vi "Resize Image (WxH).vi"(7 "Filter (Default)":T1, 8 "error in (no error)":errorcluster, 9 "Height":i32, 10 "Width":i32, 11 "Image":T2) -> (0 "error out":errorcluster, 3 "Resized Image":T2)   [LabVIEW 2020, in "G-Image.lvlib"]
doc: "Resize the input image to the specified width and height.\n\n<b>Filter</b> sets the filter type used when resizing. When set to Default, the Catmull-Rom filter is used when upsampling images, and the Mitchell filter used when downsampling images.\n\n<b>Note:</b> 8-bit images will be converted to true color images when resized."
uses:
  G-Image.lvlib
  <vilib>/picture/picture.llb/imagedata.ctl
  Controls/Resize Filter.ctl
  <vilib>/Utility/error.llb/Error Cluster From Error Code.vi
  lib/g_image_32.dll
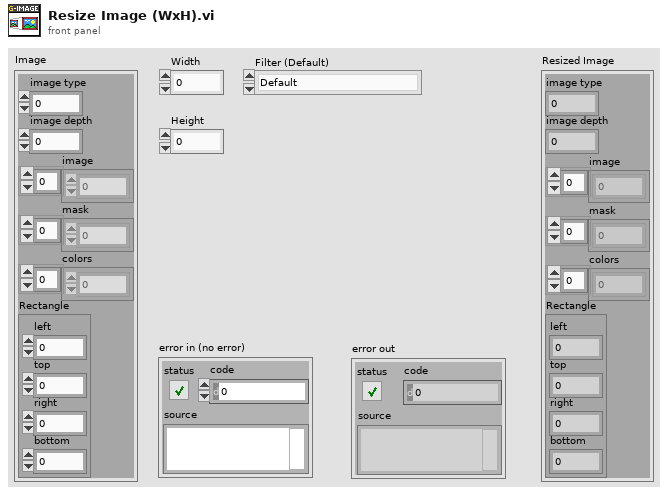
[diagram p1: front panel]
types:
  T1 = typedef "G-Image.lvlib/Resize Filter.ctl" = enum16{"Default", "Box", "Triangle", "Cubic B-Spline", "Catmull-Rom", "Mitchell"}
  T2 = typedef "imagedata.ctl" = cluster{"image type":i32, "image depth":i32, "image":u8[], "mask":u8[], "colors":u32[], "Rectangle":cluster{"left":i16, "top":i16, "right":i16, "bottom":i16}}
  T3 = cluster{"left":i16, "top":i16, "right":i16, "bottom":i16}
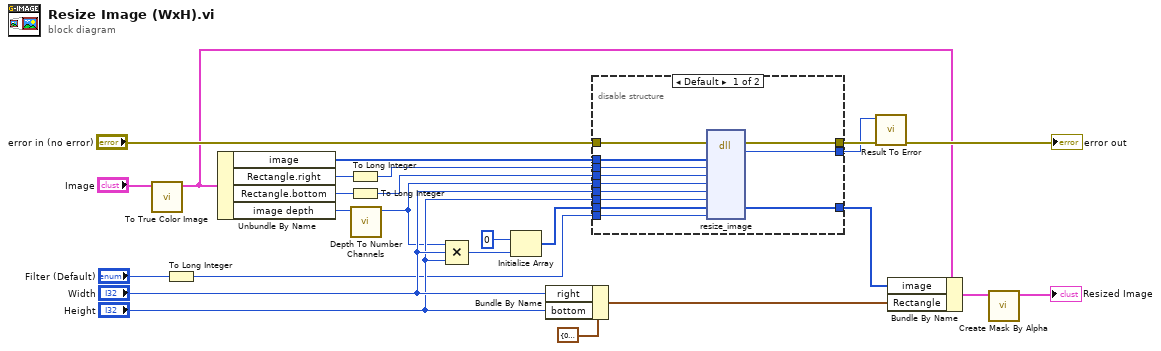
[diagram p0: block diagram]
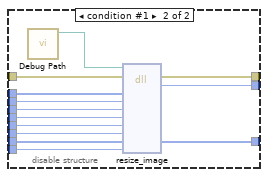
[diagram p2: hidden frame]
diagram:
  n1 = call "To True Color Image.vi"("Image"="Image") -> ("True Color Image"=w3:T2)  [unwired: 9 in, 1 out]
  n2 = To Long Integer(number="Filter (Default)") -> (32bit integer=w1:i32)
  n3 = Unbundle By Name(w3) -> ("image"=w25:u8[], "Rectangle.right"=w12:i16, "Rectangle.bottom"=w10:i16, "image depth"=w6:i32)
  n4 = To Long Integer(number=w12) -> (32bit integer=w11:i32)
  n5 = To Long Integer(number=w10) -> (32bit integer=w9:i32)
  n6 = call "Depth To Number Channels.vi"("Depth"=w6) -> ("Channels"=w5:i32)  [unwired: 10 in]
  n7 = Compound Arithmetic op=MULTIPLY(w5, "Width", "Height") -> (w23:i32)
  n8 = Initialize Array(u8 0, w23) -> (w15:u8[])
  n9 = Bundle By Name(cluster=T3 {"left"=0, "top"=0, "right"=0, "bottom"=0} ("Rectangle"), "right"="Width", "bottom"="Height") -> (w19:T3)
  n10 = disable-structure shown="Default" {
    disable-tunnel: [w37 w50] -> w18
    disable-tunnel: "error in (no error)" -> [w36 w49]
    disable-tunnel: [w35 w48] -> w17
    disable-tunnel: w25 -> [w34 w47]
    disable-tunnel: w11 -> [w33 w46]
    disable-tunnel: w9 -> [w32 w45]
    disable-tunnel: w5 -> [w31 w44]
    disable-tunnel: "Width" -> [w30 w43]
    disable-tunnel: "Height" -> [w29 w42]
    disable-tunnel: w15 -> [w28 w41]
    disable-tunnel: [w27 w40] -> w14
    disable-tunnel: w1 -> [w26 w38]
    frame condition #0 (active) {
      n11 = dll-call lib="C:/github/dataflowg/g-image/src/LabVIEW/G-Image/lib/g_image_*.*" fn="resize_image"(error in=w36, "image_data_in"=w34, "width_in"=w33, "height_in"=w32, "channels_in"=w31, "width_resize"=w30, "height_resize"=w29, "image_data_out"=w28, "filter"=w26) -> (error out=w37:errorcluster, "result"=w35:i32, "image_data_out"=w27:u8[])  [unwired: 9 in, 1 out]
    }
    frame condition #1 {
      n12 = call "Debug Path.vi"() -> ("Debug Path"=w39:path)  [unwired: 11 in]
      n13 = dll-call lib="?" fn="resize_image"(path in=w39, error in=w49, "image_data_in"=w47, "width_in"=w46, "height_in"=w45, "channels_in"=w44, "width_resize"=w43, "height_resize"=w42, "image_data_out"=w41, "filter"=w38) -> (error out=w50:errorcluster, "result"=w48:i32, "image_data_out"=w40:u8[])  [unwired: 8 in, 1 out]
    }
  }
  n14 = call "Result To Error.vi"("error in (no error)"=w18, "Result Code"=w17) -> ("error out"=→"error out":errorcluster)  [unwired: 9 in]
  n15 = Bundle By Name(cluster=w3, "image"=w14, "Rectangle"=w19) -> (w8:T2)
  n16 = call <vilib>:"Create Mask By Alpha.vi"("image data"=w8) -> ("masked image data"=→"Resized Image":T2)  [unwired: 10 in]
